vi "Get Localized Phrase Compact Interface 0D.vi"(1 "Key":string) -> (0 "Translated Phrase":string)   [LabVIEW 2020]
doc: "Gets the localized phrase by key from the current dictionary.\n\nKey: Unique identifier defined in the dictionary\nTarget Language (current lang): Optional input. Set this to translate a phase to a language other than the current language."
uses:
  Localization FGV Action -- Enum.ctl
panel:
  out "error out":errorcluster
  in  "error in":errorcluster
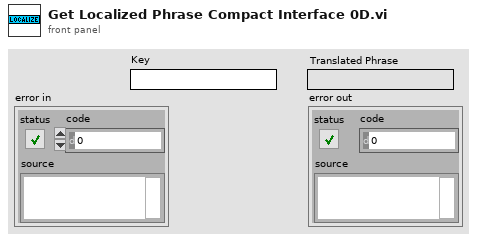
[diagram p1: front panel]
types:
  T1 = typedef "Localization FGV Action -- Enum.ctl" = enum16{"Read Dictionary", "Translate VIs", "Register VI", "Get Languages", "Translate Phrase", "Get Key For Phrase", "Get Phrase For Phrase", "Translate VI", "Unregister"}
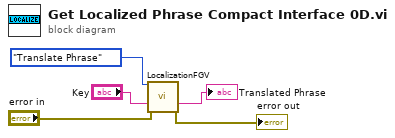
[diagram p0: block diagram]
diagram:
  n1 = call "LocalizationFGV.vi"("Action"=Localization_FGV_Action_--_Enum."Translate Phrase", "Input"="Key", "error in"="error in") -> ("Result"=→"Translated Phrase":string, "error out"=→"error out":errorcluster)  [unwired: 7 in, 4 out]
